vi "example_msgUserEventStopMechanism.vi"() -> ()   [LabVIEW 2023]
doc: "TLC Daemon Example Message User Event Stop Mechanism."
uses:
  TaskController/TaskController.lvclass
  <vilib>/numeric/Random Number (Range) U64.vi
  <vilib>/numeric/sub_Random U32.vi
  ExampleTask_MsgUserEventStop/ExampleTask_MsgUserEventStop.lvclass
panel:
  in  "sendMessage":bool
  out "error":errorcluster
  in  "stop":bool
  in  "launchNewTask":bool
  # "Example of TaskController with Message User Event Stop Mechanism"
  # "Instruction: \n1. Press RUN button.\n \n2. Press LAUNCH NEW TASK button to launch a new task \n\n3. Press SEND MESSAGE button to send a random message using the same Message User Event used by the Stop Mechanism.\n\n4. Press STOP button to stop all the active tasks using the Message User Event Stop Mechanism\n\nFor details, view code and its comments"
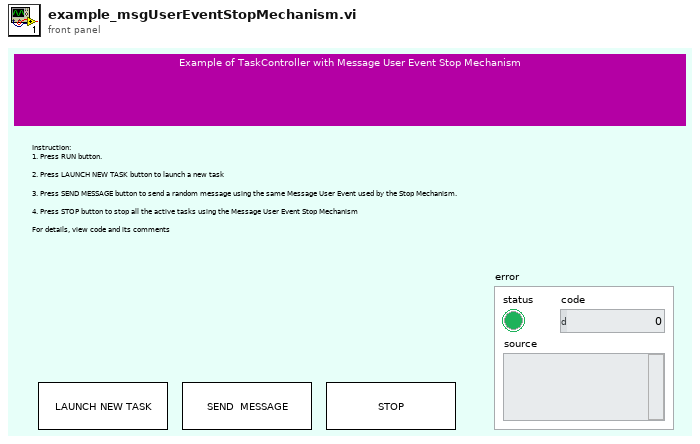
[diagram p1: front panel]
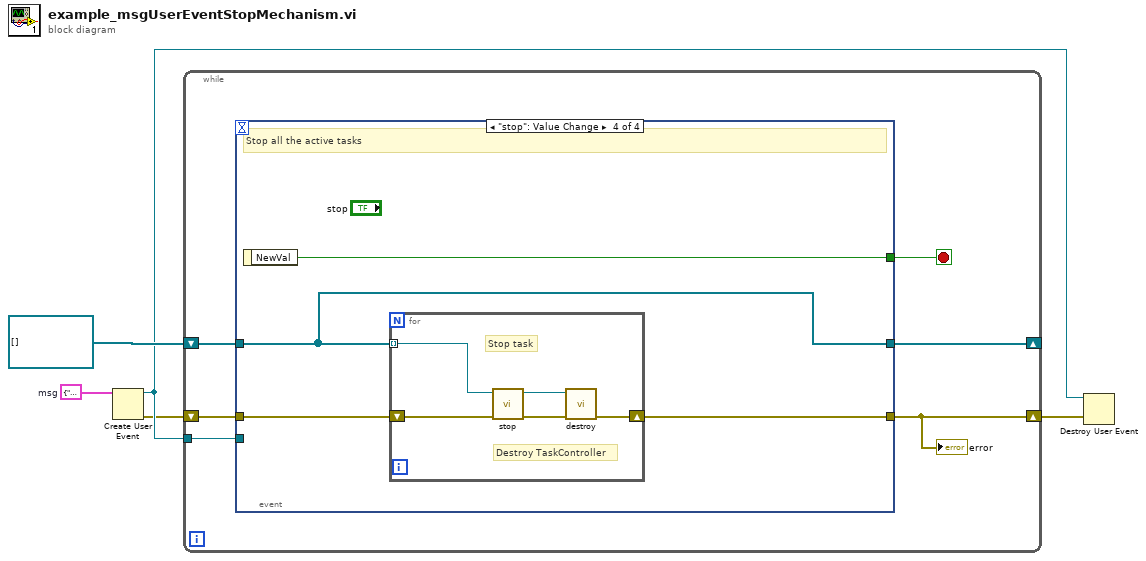
[diagram p0: block diagram]
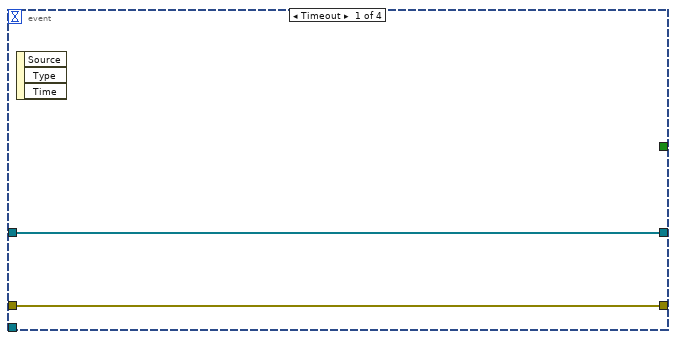
[diagram p2: hidden frame]
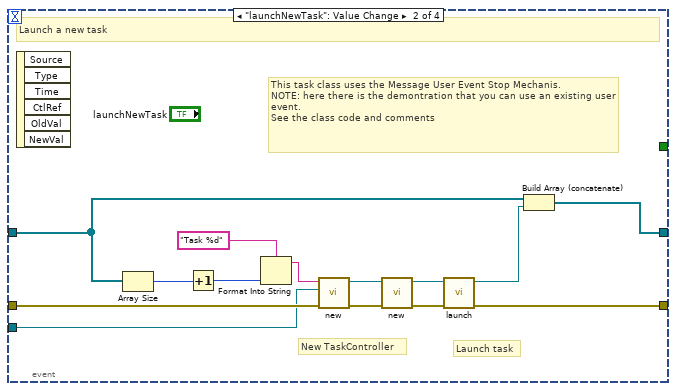
[diagram p3: hidden frame]
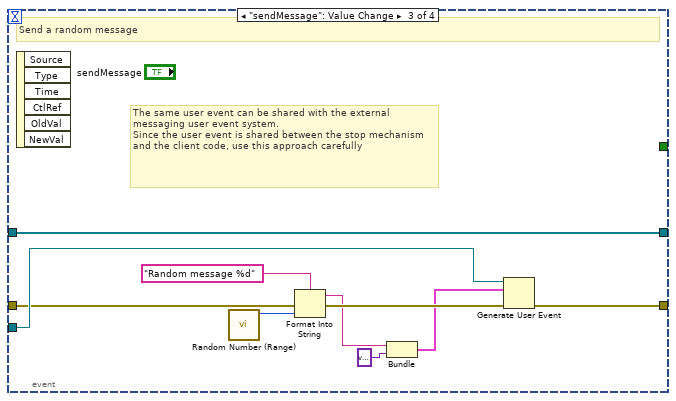
[diagram p4: hidden frame]
diagram:
  w4 = cluster{"message":string, "data":variant} {"message"="", "data"=variant}  # msg
  n1 = Create User Event(user event datatype=w4) -> (user event=w2:refnum<user-event>, error out=w1:errorcluster)  [unwired: 1 in]
  n2 = while {
    shift-right: [w11] -> _
    shift-left: refnum<class "TaskController.lvclass">[] [] -> [w10]
    shift-right: [w7] -> w3
    shift-left: w1 -> [w9]
    tunnel: w2 -> [w6]
    stop <- w8 stop-if-true
    n3 = event shown="[3] \"stop\": Value Change" {
      selector: _ -> [_ _ _ _]
      dyn-events: _ -> [_ _ _ _]
      timeout: _ -> [_ _ _ _]
      tunnel: [w13 w24 w28 w38] -> w11
      tunnel: w10 -> [w13 w22 w28 w38]
      tunnel: [w12 w23 w32 w40] -> w7
      tunnel: w9 -> [w12 w17 w34 w41]
      tunnel: [_ _ _ w39] -> w8
      tunnel: w6 -> [_ w14 w35 _]
      event Timeout {
        n4 = event-data() -> ()  [unwired: 1 in, 3 out]
      }
      event "launchNewTask": Value Change {
        # "This task class uses the Message User Event Stop Mechanis.\nNOTE: here there is the demontration that you can use an existing user event.\nSee the class code and comments"
        # "New TaskController"
        # "Launch task"
        # "Launch a new task"
        n5 = event-data() -> ()  [unwired: 1 in, 6 out]
        n6 = Array Size(array=w22) -> (size(s)=w19:i32)
        n7 = Increment(x=w19) -> (x+1=w21:i32)
        n8 = Format Into String(format string="Task %d", w21) -> (resulting string=w18:string)  [unwired: 2 in, 1 out]
        n9 = call "new.vi"("error in (no error)"=w17, "messageIn"=w14, "description"=w18) -> ("error out"=w16:errorcluster, "ExampleTask_MsgUserEventStopNotifier Out"=w15:refnum<class "ExampleTask_MsgUserEventStop.lvclass">)  [unwired: 7 in]
        n10 = call "new.vi"("error in (no error)"=w16, "task"=w15) -> ("error out"=w27:errorcluster, "TaskController out"=w26:refnum<class "TaskController.lvclass">)  [unwired: 8 in]
        n11 = call "launch.vi"("error in (no error)"=w27, "TaskController in"=w26) -> ("error out"=w23:errorcluster, "TaskController out"=w25:refnum<class "TaskController.lvclass">)  [unwired: 8 in]
        n12 = Build Array (concatenate)(w22, w25) -> (w24:refnum<class "TaskController.lvclass">[])
      }
      event "sendMessage": Value Change {
        # "The same user event can be shared with the external messaging user event system.\nSince the user event is shared between the stop mechanism and the client code, use this approach carefully"
        # "Send a random message"
        n13 = event-data() -> ()  [unwired: 1 in, 6 out]
        n14 = call-poly <vilib>:"Random Number (Range).vi"() -> ("number"=w36:u64)  [unwired: 11 in]
        n15 = Format Into String(format string="Random message %d", error in=w34, w36) -> (resulting string=w31:string, error out=w33:errorcluster)  [unwired: 1 in]
        n16 = Bundle(w31, variant) -> (w30:cluster{string, variant})  [unwired: 1 in]
        n17 = Generate User Event(user event=w35, event data cluster=w30, error in=w33) -> (error out=w32:errorcluster)  [unwired: 1 in, 1 out]
      }
      event "stop": Value Change {
        # "Stop all the active tasks"
        n18 = event-data() -> ("NewVal"=w39:bool)  [unwired: 1 in]
        n19 = for {
          tunnel: w38 -> [w44] mode=indexing
          shift-right: [w42] -> w40
          shift-left: w41 -> [w43]
          # "Destroy TaskController"
          # "Stop task"
          n20 = call "stop.vi"("error in (no error)"=w43, "TaskController in"=w44) -> ("error out"=w45:errorcluster, "TaskController out"=w46:refnum<class "TaskController.lvclass">)  [unwired: 8 in]
          n21 = call "destroy.vi"("error in (no error)"=w45, "TaskController in"=w46) -> ("error out"=w42:errorcluster)  [unwired: 7 in, 2 out]
        }
      }
    }
    "error" <- w7
  }
  n22 = Destroy User Event(user event=w2, error in=w3) -> ()  [unwired: 1 out]
